vi "voltage-current-graph.vi"() -> ()   [LabVIEW 2020]
uses:
  <vilib>/Instr/_visa.llb/VISA Configure Serial Port (Instr).vi
panel:
  out "Current":dbl format="%#_6f"
  out "Voltage":dbl
  out "Ampermeter":dbl(knob) scale=0.0..5.0
  out "Voltmeter":dbl(knob) scale=0.0..30.0
  in  "Current multiplier":dbl=1.0 min=0.0
  in  "Voltage multiplier":dbl=1.0 min=0.0
  out "Voltage-current graph":dynamicdata(graph)
  in  "Sampling rate (hz)":u32=50 min=1
  in  "COM Port":refnum<visa-resource-name>
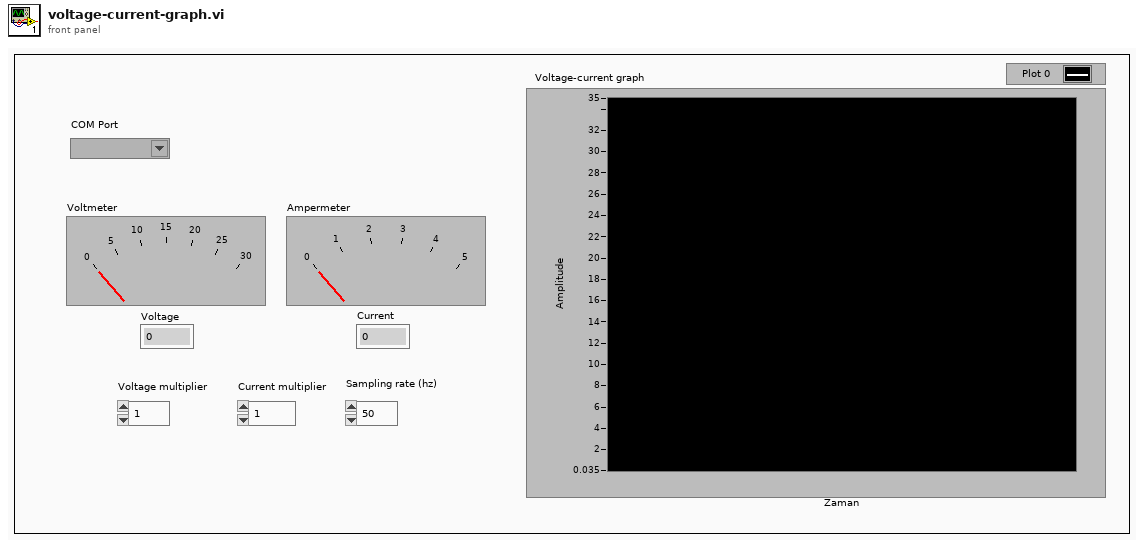
[diagram p1: front panel]
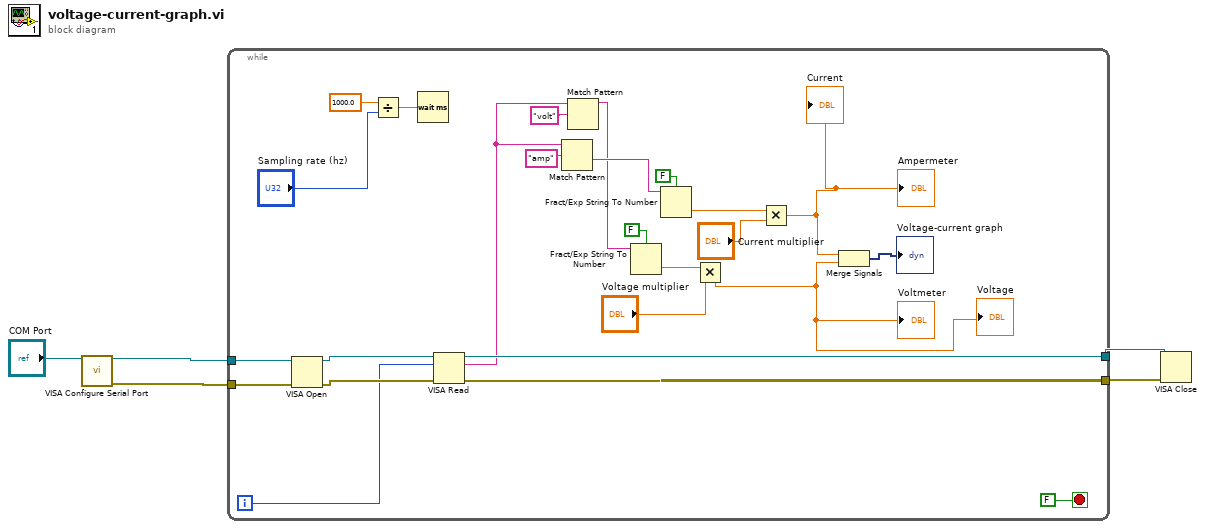
[diagram p0: block diagram]
diagram:
  n1 = call-poly "VISA Configure Serial Port"("VISA resource name"="COM Port") -> ("VISA resource name out"=w1:refnum<visa-resource-name>, "error out"=w2:errorcluster)  [unwired: 13 in]
  n2 = while {
    tunnel: w2 -> [w30]
    tunnel: [w28] -> w5
    tunnel: w1 -> [w27]
    tunnel: [w25] -> w4
    i -> [w24]
    stop <- FALSE stop-if-true
    n3 = VISA Open(error in (no error)=w30, VISA resource name=w27) -> (VISA resource name=w26:refnum<visa-resource-name>, error out=w29:errorcluster)  [unwired: 3 in]
    n4 = Divide(x=1000.0, y="Sampling rate (hz)") -> (x/y=w9:dbl)
    n5 = Wait (ms)(milliseconds to wait=w9) -> ()  [unwired: 1 out]
    n6 = VISA Read(VISA resource name=w26, byte count=w24, error in (no error)=w29) -> (VISA resource name out=w25:refnum<visa-resource-name>, read buffer=w20:string, error out=w28:errorcluster)  [unwired: 1 out]
    n7 = Match Pattern(string=w20, regular expression="amp") -> (after substring=w19:string)  [unwired: 1 in, 3 out]
    n8 = Match Pattern(string=w20, regular expression="volt") -> (before substring=w8:string)  [unwired: 1 in, 3 out]
    n9 = Fract/Exp String To Number(use system decimal point (T)=FALSE, string=w8) -> (number=w15:dbl)  [unwired: 2 in, 1 out]
    n10 = Fract/Exp String To Number(use system decimal point (T)=FALSE, string=w19) -> (number=w13:dbl)  [unwired: 2 in, 1 out]
    n11 = Multiply(x=w15, y="Voltage multiplier") -> (x*y=w7:dbl)
    "Voltmeter" <- w7
    "Voltage" <- w7
    n12 = Multiply(x=w13, y="Current multiplier") -> (x*y=w6:dbl)
    "Ampermeter" <- w6
    "Current" <- w6
    n13 = Merge Signals(w6, w7) -> (→"Voltage-current graph":dynamicdata)
  }
  n14 = VISA Close(VISA resource name=w4, error in (no error)=w5) -> ()  [unwired: 1 out]
